vi "destroyTempControllerBackEndEvents.vi"(8 "error in (no error)":errorcluster, 10 "tempControllerBackEndEvents":T1, 11 "CameraEventsManger in":refnum<class "CameraEventsManger.lvclass">) -> (0 "error out":errorcluster, 3 "CameraEventsManger out":refnum<class "CameraEventsManger.lvclass">)   [LabVIEW 2011, in "Tools.lvlib" / "Settings.lvlib" / "CameraEventsManger.lvclass"]
uses:
  CameraEventsManger.lvclass
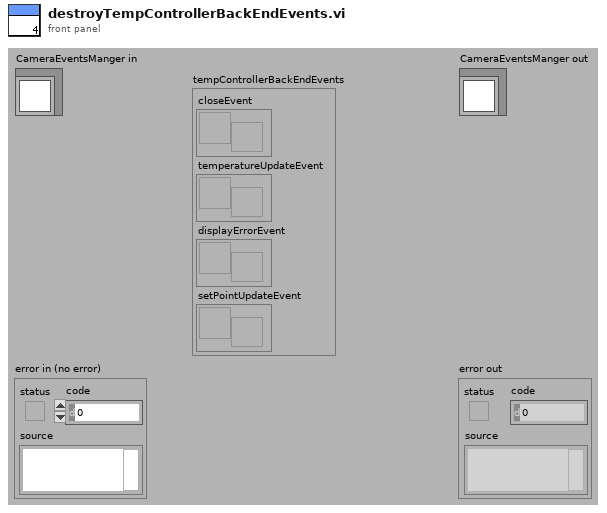
[diagram p1: front panel]
types:
  T1 = cluster{"closeEvent":refnum<user-event>, "temperatureUpdateEvent":refnum<user-event>, "displayErrorEvent":refnum<user-event>, "setPointUpdateEvent":refnum<user-event>}
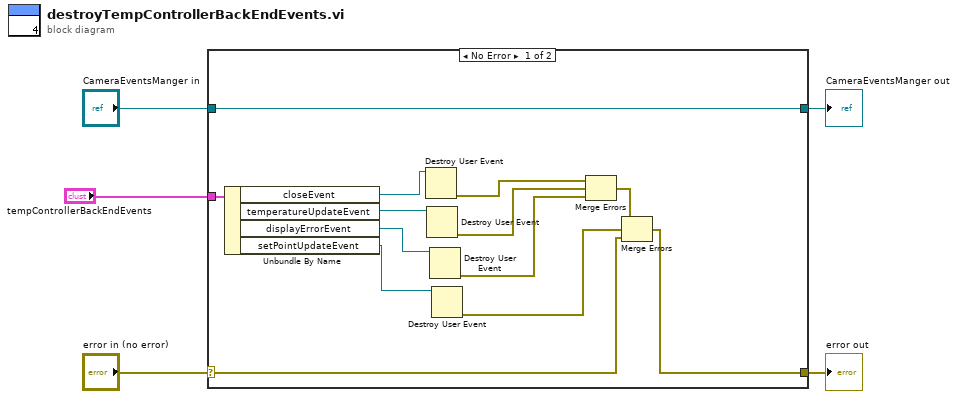
[diagram p0: block diagram]
diagram:
  n1 = case shown="No Error" "error in (no error)" {
    selector: "error in (no error)" -> [w6 w20]
    tunnel: [w7 w20] -> w4
    tunnel: [w18 w19] -> w2
    tunnel: "CameraEventsManger in" -> [w18 w19]
    tunnel: "tempControllerBackEndEvents" -> [w17 _]
    frame No Error {
      n2 = Unbundle By Name(w17) -> ("closeEvent"=w16:refnum<user-event>, "temperatureUpdateEvent"=w15:refnum<user-event>, "displayErrorEvent"=w14:refnum<user-event>, "setPointUpdateEvent"=w13:refnum<user-event>)
      n3 = Destroy User Event(user event=w16) -> (error out=w12:errorcluster)  [unwired: 1 in]
      n4 = Destroy User Event(user event=w15) -> (error out=w11:errorcluster)  [unwired: 1 in]
      n5 = Destroy User Event(user event=w14) -> (error out=w10:errorcluster)  [unwired: 1 in]
      n6 = Destroy User Event(user event=w13) -> (error out=w8:errorcluster)  [unwired: 1 in]
      n7 = Merge Errors(w12, w11, w10) -> (w9:errorcluster)
      n8 = Merge Errors(w9, w8, w6) -> (w7:errorcluster)
    }
    frame Error {
    }
  }
  "error out" <- w4
  "CameraEventsManger out" <- w2
